vi "AD_Single.vi"() -> ()   [LabVIEW 2012]
uses:
  Usb_Daq_V52_Dll.dll
panel:
  out "AD 8":dbl
  out "AD 7":dbl
  out "AD 6":dbl
  out "AD 5":dbl
  out "AD 4":dbl
  out "AD 3":dbl
  out "AD 2":dbl
  out "AD1":dbl
  in  "stop":bool
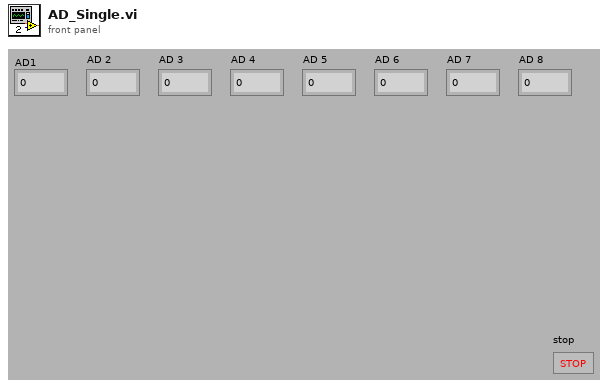
[diagram p1: front panel]
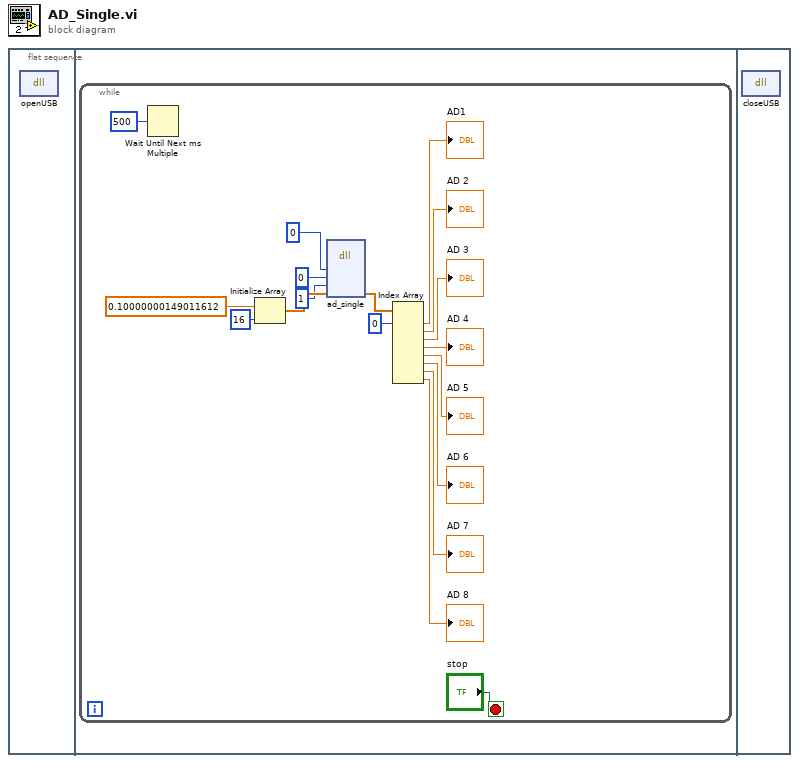
[diagram p0: block diagram]
diagram:
  n1 = flat-sequence {
    frame #0 {
      n2 = dll-call lib="PTH1labs Ebackup数据采集卡uSB!USB数据采集卡资料HKUSB6203例程labviewUsb_Daq_V52_Dll.dll" fn="openUSB"() -> ()  [unwired: 3 in, 3 out]
    }
    frame #1 {
      n3 = while {
        stop <- "stop" stop-if-true
        n4 = Wait Until Next ms Multiple(millisecond multiple=500) -> ()  [unwired: 1 out]
        n5 = Initialize Array(sgl 0.1, 16) -> (w14:sgl[])
        n6 = dll-call lib="PTH1labs Ebackup数据采集卡uSB!USB数据采集卡资料HKUSB6203例程labviewUsb_Daq_V52_Dll.dll" fn="ad_single"("dev"=0, "Over_Sample"=0, "gain"=1, "result"=w14) -> ("result"=w11:sgl[])  [unwired: 7 in, 2 out]
        n7 = Index Array(array=w11, index #1=0) -> (element #1=→"AD1":sgl, element #2=→"AD 2":sgl, element #3=→"AD 3":sgl, element #4=→"AD 4":sgl, element #5=→"AD 5":sgl, element #6=→"AD 6":sgl, element #7=→"AD 7":sgl, element #8=→"AD 8":sgl)  [unwired: 7 in]
      }
    }
    frame #2 {
      n8 = dll-call lib="PTH1labs Ebackup数据采集卡uSB!USB数据采集卡资料HKUSB6203例程labviewUsb_Daq_V52_Dll.dll" fn="closeUSB"() -> ()  [unwired: 3 in, 3 out]
    }
  }
